vi "Filter Properties.vi"(8 "error in":errorcluster, 11 "Data":T1) -> (0 "error out":errorcluster, 3 "Data Out":T1)   [LabVIEW 2014]
uses:
  Controls/Data.ctl
  Controls/FP Control Refs.ctl
  Controls/Property.ctl
  Controls/Address.ctl
  Controls/Filter Criteria.ctl
  Controls/Fields.ctl
  Controls/Operator.ctl
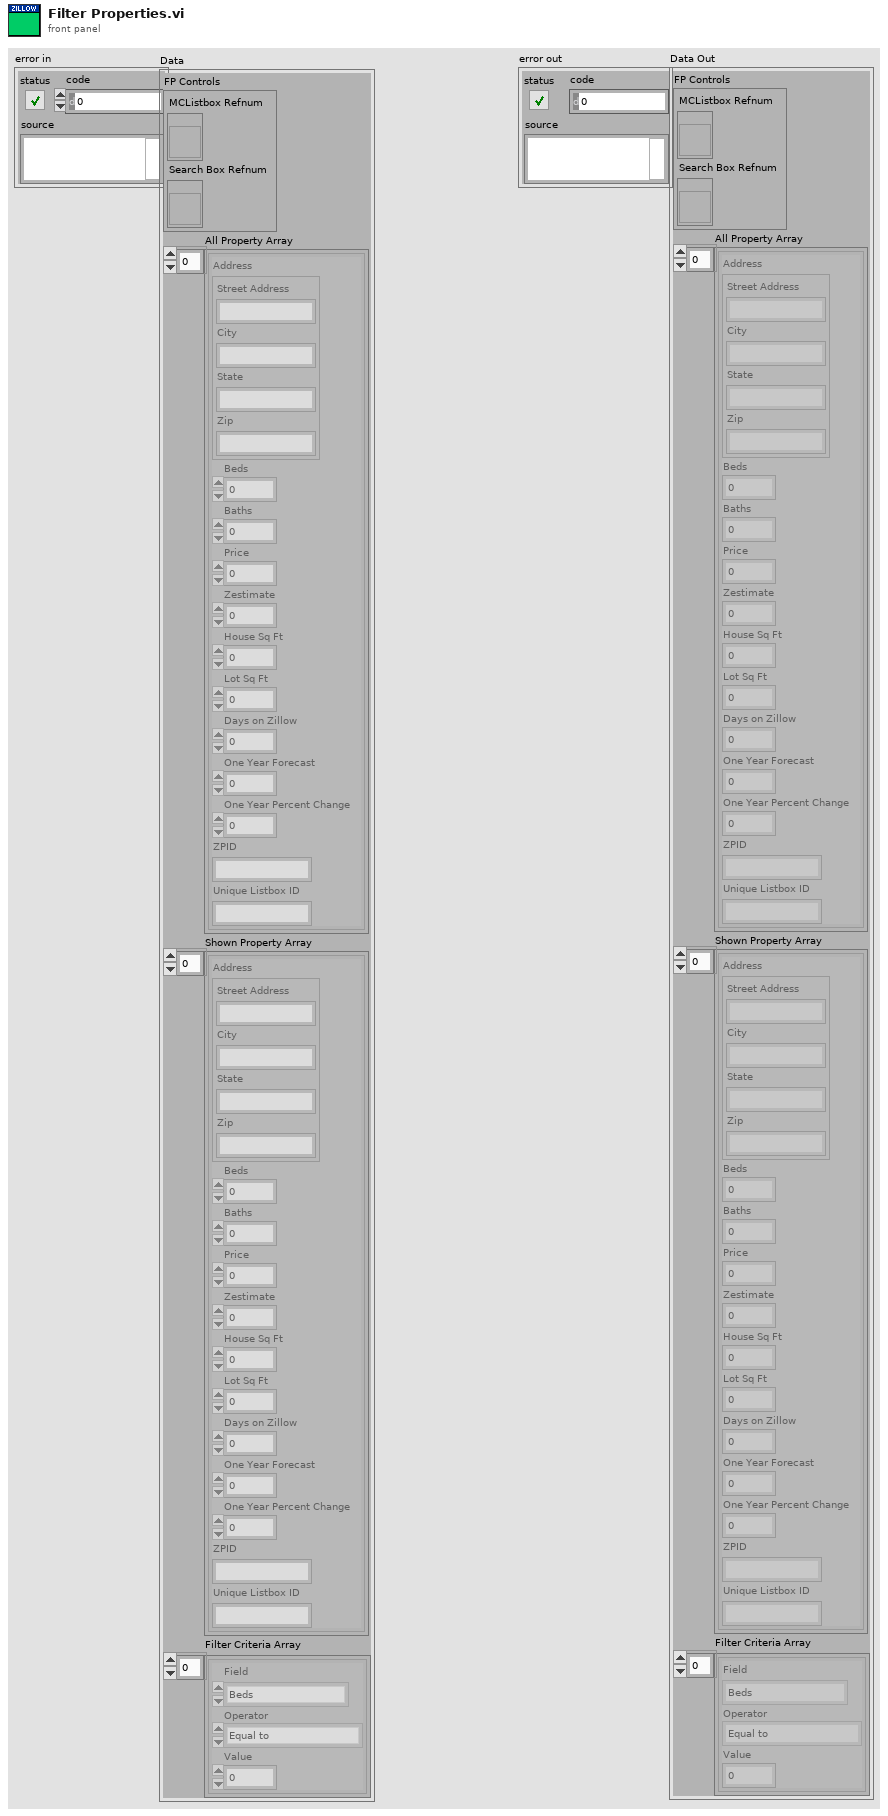
[diagram p1: front panel]
types:
  T1 = typedef "Data.ctl" = cluster{"FP Controls":T2, "All Property Array":T3[], "Shown Property Array":T3[], "Filter Criteria Array":T5[]}
  T2 = typedef "FP Control Refs.ctl" = cluster{"MCListbox Refnum":refnum<vi>, "Search Box Refnum":refnum<vi>}
  T3 = typedef "Property.ctl" = cluster{"Address":T4, "Beds":dbl, "Baths":dbl, "Price":dbl, "Zestimate":dbl, "House Sq Ft":dbl, "Lot Sq Ft":dbl, "Days on Zillow":dbl, "One Year Forecast":dbl, "One Year Percent Change":dbl, "ZPID":string, "Unique Listbox ID":string}
  T4 = typedef "Address.ctl" = cluster{"Street Address":string, "City":string, "State":string, "Zip":string}
  T5 = typedef "Filter Criteria.ctl" = cluster{"Field":T6, "Operator":T7, "Value":dbl}
  T6 = typedef "Fields.ctl" = enum16{"Beds", "Baths", "Price", "Zestimate", "House Sq Ft", "Lot Sq Ft", "Days on Zillow", "One Year Forecast", "One Year Percent Change"}
  T7 = typedef "Operator.ctl" = enum16{"Equal to", "Greater than (or equal)", "Less than (or equal)", "Not Equal to"}
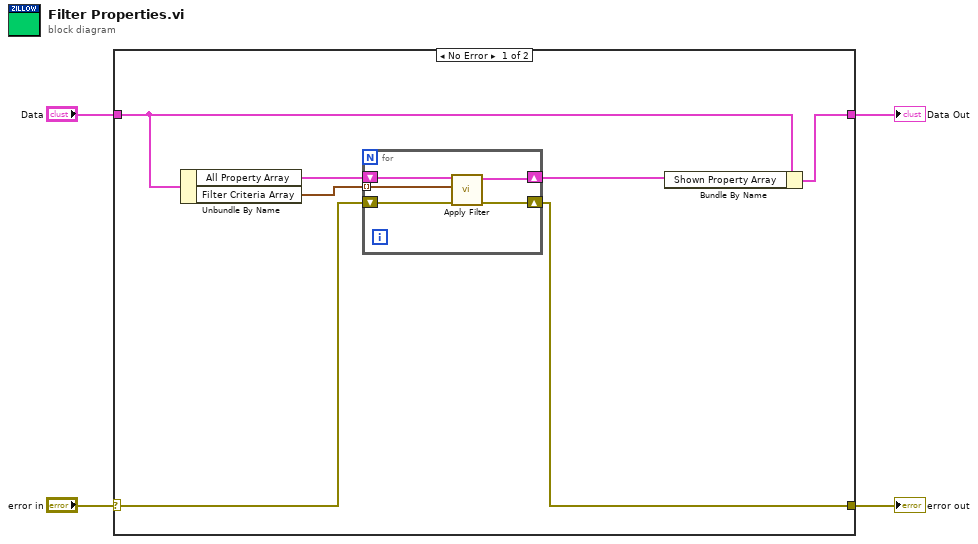
[diagram p0: block diagram]
diagram:
  n1 = case shown="No Error" "error in" {
    selector: "error in" -> [w6 w18]
    tunnel: [w5 w18] -> w3
    tunnel: "Data" -> [w11 w17]
    tunnel: [w10 w17] -> w1
    frame No Error {
      n2 = Unbundle By Name(w11) -> ("All Property Array"=w9:T3[], "Filter Criteria Array"=w8:T5[])
      n3 = for {
        tunnel: w8 -> [w15] mode=indexing
        shift-right: [w14] -> w7
        shift-left: w9 -> [w16]
        shift-right: [w12] -> w5
        shift-left: w6 -> [w13]
        n4 = call "Apply Filter.vi"("error in"=w13, "Filter Criteria"=w15, "Property Array"=w16) -> ("error out"=w12:errorcluster, "Filtered Property Array Out"=w14:T3[])  [unwired: 7 in]
      }
      n5 = Bundle By Name(cluster=w11, "Shown Property Array"=w7) -> (w10:T1)
    }
    frame Error {
    }
  }
  "error out" <- w3
  "Data Out" <- w1
